vi "EnFlo_TubingCorrection.vi"() -> ()   [LabVIEW 2022 SP3]
uses:
  Globals/Meas_global.vi
  <vilib>/Analysis/NI_AALBase.lvlib
  <vilib>/Analysis/baseanly.llb/Mean (DBL).vi
  <vilib>/gmath/NI_Gmath.lvlib
  Controls/Setup.ctl
panel:
  in  "Correlation Mode":T1(ring)
  in  "Desired Freq Hz":sgl=80.0
  out "Averaging samples":i32=5
  in  "Switch off Tubing Correction?":bool
  out "Correlation Coefficients":string[][](table)
  out "?":dbl[](graph)
  in  "Subtract Mode":T2(ring)
  in  "Reference Instrument":i32(ring) items=["None", "RZ (C0_P00):COM30_Ch 0", "RZ (C0_P01):COM30_Ch 1", "RZ (C0_P02):COM30_Ch 2", "RZ (C0_P03):COM30_Ch 3", "RZ (C0_P04):COM30_Ch 4", "RZ (C0_P05):COM30_Ch 5", "RZ (C0_P06):COM30_Ch 6", "RZ (C0_P07):COM30_Ch 7", "RZ (C0_P10):COM30_Ch 8", "RZ (C0_P11):COM30_Ch 9", "RZ (C0_P12):COM30_Ch 10", "RZ (C0_P13):COM30_Ch 11", "RZ (C0_P14):COM30_Ch 12", "RZ (C0_P15):COM30_Ch 13", "RZ (C0_P16):COM30_Ch 14", "RZ (C0_P17):COM30_Ch 15", "RZ (C0_P20):COM30_Ch 16", "RZ (C0_P21):COM30_Ch 17", "RZ (C0_P22):COM30_Ch 18", "RZ (C0_P23):COM30_Ch 19", "RZ (C0_P24):COM30_Ch 20", "RZ (C0_P25):COM30_Ch 21", "RZ (C0_P26):COM30_Ch 22", "RZ (C0_P27):COM30_Ch 23", "RZ (C0_P30):COM30_Ch 24", "RZ (C0_P31):COM30_Ch 25", "RZ (C0_P32):COM30_Ch 26", "RZ (C0_P33):COM30_Ch 27", "RZ (C0_P34):COM30_Ch 28", "RZ (C0_P35):COM30_Ch 29", "RZ (C0_P36):COM30_Ch 30", "RZ (C0_P37):COM30_Ch 31", "RZ (C0_P40):COM30_Ch 32", "RZ (C0_P41):COM30_Ch 33", "RZ (C0_P42):COM30_Ch 34", "RZ (C0_P43):COM30_Ch 35", "RZ (C0_P44):COM30_Ch 36", "RZ (C0_P45):COM30_Ch 37", "RZ (C0_P46):COM30_Ch 38", "RZ (C0_P47):COM30_Ch 39", "RZ (C0_P50):COM30_Ch 40", "RZ (C0_P51):COM30_Ch 41", "RZ (C1_P73):COM31_Ch 59", "RZ (C0_P53):COM30_Ch 43", "RZ (C0_P54):COM30_Ch 44", "RZ (C0_P55):COM30_Ch 45", "RZ (C0_P56):COM30_Ch 46", "RZ (C0_P57):COM30_Ch 47", "RZ (C0_P60):COM30_Ch 48", "RZ (C0_P62):COM30_Ch 50", "RZ (C0_P63):COM30_Ch 51", "RZ (C0_P64):COM30_Ch 52", "RZ (C0_P65):COM30_Ch 53", "RZ (C0_P66):COM30_Ch 54", "RZ (C0_P67):COM30_Ch 55", "RZ (C0_P70):COM30_Ch 56", "RZ (C0_P71):COM30_Ch 57", "RZ (C0_P72):COM30_Ch 58", "RZ (C0_P73):COM30_Ch 59", "RZ (C0_P74):COM30_Ch 60", "RZ (C0_P75):COM30_Ch 61", "RZ (C0_P76):COM30_Ch 62", "RZ (C0_P77):COM30_Ch 63", "RZ (C1_P00):COM31_Ch 0", "RZ (C1_P01):COM31_Ch 1", "RZ (C1_P02):COM31_Ch 2", "RZ (C1_P03):COM31_Ch 3", "RZ (C1_P04):COM31_Ch 4", "RZ (C1_P05):COM31_Ch 5", "RZ (C1_P06):COM31_Ch 6", "RZ (C1_P07):COM31_Ch 7", "RZ (C1_P10):COM31_Ch 8", "RZ (C1_P11):COM31_Ch 9", "RZ (C1_P12):COM31_Ch 10", "RZ (C1_P13):COM31_Ch 11", "RZ (C1_P14):COM31_Ch 12", "RZ (C1_P15):COM31_Ch 13", "RZ (C1_P16):COM31_Ch 14", "RZ (C1_P17):COM31_Ch 15", "RZ (C1_P20):COM31_Ch 16", "RZ (C1_P21):COM31_Ch 17", "RZ (C1_P22):COM31_Ch 18", "RZ (C1_P23):COM31_Ch 19", "RZ (C1_P24):COM31_Ch 20", "RZ (C1_P25):COM31_Ch 21", "RZ (C1_P26):COM31_Ch 22", "RZ (C1_P27):COM31_Ch 23", "RZ (C1_P30):COM31_Ch 24", "RZ (C1_P31):COM31_Ch 25", "RZ (C1_P32):COM31_Ch 26", "RZ (C1_P33):COM31_Ch 27", "RZ (C1_P34):COM31_Ch 28", "RZ (C1_P35):COM31_Ch 29", "RZ (C1_P36):COM31_Ch 30", "RZ (C1_P37):COM31_Ch 31", "RZ (C1_P40):COM31_Ch 32", "RZ (C1_P41):COM31_Ch 33", "RZ (C1_P42):COM31_Ch 34", "RZ (C1_P43):COM31_Ch 35", "RZ (C1_P44):COM31_Ch 36", "RZ (C1_P45):COM31_Ch 37", "RZ (C1_P46):COM31_Ch 38", "RZ (C1_P47):COM31_Ch 39", "RZ (C1_P50):COM31_Ch 40", "RZ (C1_P51):COM31_Ch 41", "RZ (C1_P52):COM31_Ch 42", "RZ (C1_P53):COM31_Ch 43", "RZ (C1_P54):COM31_Ch 44", "RZ (C1_P55):COM31_Ch 45", "RZ (C1_P56):COM31_Ch 46", "RZ (C1_P57):COM31_Ch 47", "RZ (C1_P60):COM31_Ch 48", "RZ (C1_P61):COM31_Ch 49", "RZ (C1_P62):COM31_Ch 50", "RZ (C1_P63):COM31_Ch 51", "RZ (C2_P00):COM33_Ch 0", "RZ (C2_P01):COM33_Ch 1", "RZ (C2_P02):COM33_Ch 2", "RZ (C2_P03):COM33_Ch 3", "RZ (C2_P04):COM33_Ch 4", "RZ (C2_P05):COM33_Ch 5", "RZ (C2_P06):COM33_Ch 6", "RZ (C2_P07):COM33_Ch 7", "RZ (C2_P10):COM33_Ch 8", "RZ (C2_P11):COM33_Ch 9", "RZ (C2_P12):COM33_Ch 10", "RZ (C2_P13):COM33_Ch 11", "RZ (C2_P14):COM33_Ch 12", "RZ (C2_P15):COM33_Ch 13", "RZ (C2_P16):COM33_Ch 14", "RZ (C2_P17):COM33_Ch 15", "RZ (C2_P20):COM33_Ch 16", "RZ (C2_P21):COM33_Ch 17", "RZ (C2_P22):COM33_Ch 18", "RZ (C2_P23):COM33_Ch 19", "RZ (C2_P24):COM33_Ch 20", "RZ (C2_P25):COM33_Ch 21", "RZ (C2_P26):COM33_Ch 22", "RZ (C2_P27):COM33_Ch 23", "RZ (C2_P31):COM33_Ch 25", "RZ (C2_P32):COM33_Ch 26", "RZ (C2_P33):COM33_Ch 27", "RZ (C2_P34):COM33_Ch 28", "RZ (C2_P35):COM33_Ch 29", "RZ (C2_P36):COM33_Ch 30", "RZ (C2_P37):COM33_Ch 31", "RZ (C2_P40):COM33_Ch 32", "RZ (C2_P41):COM33_Ch 33", "RZ (C2_P42):COM33_Ch 34", "RZ (C2_P43):COM33_Ch 35", "RZ (C2_P44):COM33_Ch 36", "RZ (C2_P45):COM33_Ch 37", "RZ (C2_P46):COM33_Ch 38", "RZ (C2_P47):COM33_Ch 39", "RZ (C2_P50):COM33_Ch 40", "RZ (C2_P51):COM33_Ch 41", "RZ (C2_P52):COM33_Ch 42", "RZ (C2_P53):COM33_Ch 43", "RZ (C2_P54):COM33_Ch 44", "RZ (C2_P55):COM33_Ch 45", "RZ (C2_P56):COM33_Ch 46", "RZ (C2_P57):COM33_Ch 47", "RZ (C2_P60):COM33_Ch 48", "RZ (C2_P61):COM33_Ch 49", "RZ (C2_P62):COM33_Ch 50", "RZ (C2_P63):COM33_Ch 51", "RZ (C2_P64):COM33_Ch 52", "RZ (C2_P65):COM33_Ch 53", "RZ (C2_P66):COM33_Ch 54", "RZ (C2_P67):COM33_Ch 55", "RZ (C2_P70):COM33_Ch 56", "RZ (C2_P71):COM33_Ch 57", "RZ (C2_P72):COM33_Ch 58", "RZ (C2_P73):COM33_Ch 59", "RZ (C2_P74):COM33_Ch 60", "RZ (C2_P75):COM33_Ch 61", "RZ (C2_P76):COM33_Ch 62", "RZ (C2_P77):COM33_Ch 63", "RZ (C3_P00):COM32_Ch 0", "RZ (C3_P01):COM32_Ch 1", "RZ (C3_P02):COM32_Ch 2", "RZ (C3_P03):COM32_Ch 3", "RZ (C3_P04):COM32_Ch 4", "RZ (C3_P05):COM32_Ch 5", "RZ (C3_P06):COM32_Ch 6", "RZ (C3_P07):COM32_Ch 7", "RZ (C3_P10):COM32_Ch 8", "RZ (C3_P11):COM32_Ch 9", "RZ (C3_P12):COM32_Ch 10", "RZ (C3_P13):COM32_Ch 11", "RZ (C3_P14):COM32_Ch 12", "RZ (C3_P15):COM32_Ch 13", "RZ (C3_P16):COM32_Ch 14", "RZ (C3_P17):COM32_Ch 15", "RZ (C3_P20):COM32_Ch 16", "RZ (C3_P21):COM32_Ch 17", "RZ (C3_P22):COM32_Ch 18", "RZ (C3_P23):COM32_Ch 19", "RZ (C3_P24):COM32_Ch 20", "RZ (C3_P25):COM32_Ch 21", "RZ (C3_P26):COM32_Ch 22", "RZ (C3_P27):COM32_Ch 23", "RZ (C3_P30):COM32_Ch 24", "RZ (C3_P31):COM32_Ch 25", "RZ (C3_P33):COM32_Ch 27", "RZ (C3_P34):COM32_Ch 28", "RZ (C3_P35):COM32_Ch 29", "RZ (C3_P36):COM32_Ch 30", "RZ (C3_P37):COM32_Ch 31", "RZ (C3_P40):COM32_Ch 32", "RZ (C3_P41):COM32_Ch 33", "RZ (C3_P42):COM32_Ch 34", "RZ (C3_P43):COM32_Ch 35", "RZ (C3_P44):COM32_Ch 36", "RZ (C3_P45):COM32_Ch 37", "RZ (C3_P46):COM32_Ch 38", "RZ (C3_P47):COM32_Ch 39", "RZ (C3_P50):COM32_Ch 40", "RZ (C3_P51):COM32_Ch 41", "RZ (C3_P52):COM32_Ch 42", "RZ (C3_P53):COM32_Ch 43", "RZ (C3_P54):COM32_Ch 44", "RZ (C3_P55):COM32_Ch 45", "RZ (C3_P56):COM32_Ch 46", "RZ (C3_P60):COM32_Ch 48", "RZ (C3_P61):COM32_Ch 49", "RZ (C3_P62):COM32_Ch 50", "RZ (C3_P63):COM32_Ch 51", "RZ (C3_P64):COM32_Ch 52", "RZ (C3_P65):COM32_Ch 53", "RZ (C3_P66):COM32_Ch 54", "RZ (C3_P70):COM32_Ch 56", "RZ (C3_P71):COM32_Ch 57", "RZ (C3_P72):COM32_Ch 58", "RZ (C3_P73):COM32_Ch 59", "RZ (C3_P74):COM32_Ch 60", "RZ (C3_P75):COM32_Ch 61", "RZ (C3_P77):COM32_Ch 63", "RZ (C4_P00):COM25_Ch 0", "RZ (C4_P01):COM25_Ch 1", "RZ (C4_P02):COM25_Ch 2", "RZ (C4_P03):COM25_Ch 3", "RZ (C4_P04):COM25_Ch 4", "RZ (C4_P05):COM25_Ch 5", "RZ (C4_P06):COM25_Ch 6", "RZ (C4_P07):COM25_Ch 7", "RZ (C4_P10):COM25_Ch 8", "RZ (C4_P11):COM25_Ch 9", "RZ (C4_P12):COM25_Ch 10", "RZ (C4_P13):COM25_Ch 11", "RZ (C4_P15):COM25_Ch 13", "RZ (C4_P16):COM25_Ch 14", "RZ (C4_P17):COM25_Ch 15", "RZ (C4_P20):COM25_Ch 16", "RZ (C4_P21):COM25_Ch 17", "RZ (C4_P22):COM25_Ch 18", "RZ (C4_P23):COM25_Ch 19", "RZ (C4_P24):COM25_Ch 20", "RZ (C4_P26):COM25_Ch 22", "RZ (C4_P27):COM25_Ch 23", "RZ (C4_P30):COM25_Ch 24", "RZ (C4_P32):COM25_Ch 26", "RZ (C4_P33):COM25_Ch 27", "RZ (C4_P34):COM25_Ch 28", "RZ (C4_P35):COM25_Ch 29", "RZ (C4_P36):COM25_Ch 30", "RZ (C4_P37):COM25_Ch 31", "RZ (C4_P40):COM25_Ch 32", "RZ (C4_P41):COM25_Ch 33", "RZ (C4_P42):COM25_Ch 34", "RZ (C4_P43):COM25_Ch 35", "RZ (C4_P44):COM25_Ch 36", "RZ (C4_P45):COM25_Ch 37", "RZ (C4_P46):COM25_Ch 38", "RZ (C4_P47):COM25_Ch 39", "RZ (C4_P50):COM25_Ch 40", "RZ (C4_P51):COM25_Ch 41", "RZ (C4_P52):COM25_Ch 42", "RZ (C4_P53):COM25_Ch 43", "RZ (C4_P54):COM25_Ch 44", "RZ (C4_P55):COM25_Ch 45", "RZ (C4_P56):COM25_Ch 46", "RZ (C4_P57):COM25_Ch 47", "RZ (C4_P60):COM25_Ch 48", "RZ (C4_P61):COM25_Ch 49", "RZ (C4_P62):COM25_Ch 50", "RZ (C4_P63):COM25_Ch 51", "RZ (C4_P64):COM25_Ch 52", "RZ (C4_P65):COM25_Ch 53", "RZ (C4_P66):COM25_Ch 54", "RZ (C4_P67):COM25_Ch 55", "RZ (C4_P70):COM25_Ch 56", "RZ (C4_P71):COM25_Ch 57", "RZ (C4_P72):COM25_Ch 58", "RZ (C4_P73):COM25_Ch 59", "RZ (C4_P74):COM25_Ch 60", "RZ (C4_P75):COM25_Ch 61", "RZ (C4_P76):COM25_Ch 62", "RZ (C4_P77):COM25_Ch 63", "RZ (C5_P00):COM26_Ch 0", "RZ (C5_P01):COM26_Ch 1", "RZ (C5_P02):COM26_Ch 2", "RZ (C5_P03):COM26_Ch 3", "RZ (C5_P04):COM26_Ch 4", "RZ (C5_P05):COM26_Ch 5", "RZ (C5_P06):COM26_Ch 6", "RZ (C5_P07):COM26_Ch 7", "RZ (C5_P10):COM26_Ch 8", "RZ (C5_P11):COM26_Ch 9", "RZ (C5_P12):COM26_Ch 10", "RZ (C5_P13):COM26_Ch 11", "RZ (C5_P14):COM26_Ch 12", "RZ (C5_P15):COM26_Ch 13", "RZ (C5_P16):COM26_Ch 14", "RZ (C5_P17):COM26_Ch 15", "RZ (C5_P20):COM26_Ch 16", "RZ (C5_P21):COM26_Ch 17", "RZ (C5_P22):COM26_Ch 18", "RZ (C5_P23):COM26_Ch 19", "RZ (C5_P24):COM26_Ch 20", "RZ (C5_P25):COM26_Ch 21", "RZ (C5_P26):COM26_Ch 22", "RZ (C5_P27):COM26_Ch 23", "RZ (C5_P30):COM26_Ch 24", "RZ (C5_P31):COM26_Ch 25", "RZ (C5_P32):COM26_Ch 26", "RZ (C5_P33):COM26_Ch 27", "RZ (C5_P34):COM26_Ch 28", "RZ (C5_P35):COM26_Ch 29", "RZ (C5_P36):COM26_Ch 30", "RZ (C5_P37):COM26_Ch 31", "RZ (C5_P40):COM26_Ch 32", "RZ (C5_P41):COM26_Ch 33", "RZ (C5_P42):COM26_Ch 34", "RZ (C5_P43):COM26_Ch 35", "RZ (C5_P44):COM26_Ch 36", "RZ (C5_P45):COM26_Ch 37", "RZ (C5_P46):COM26_Ch 38", "RZ (C5_P47):COM26_Ch 39", "RZ (C5_P50):COM26_Ch 40", "RZ (C5_P51):COM26_Ch 41", "RZ (C5_P52):COM26_Ch 42", "RZ (C5_P53):COM26_Ch 43", "RZ (C5_P54):COM26_Ch 44", "RZ (C5_P55):COM26_Ch 45", "RZ (C5_P56):COM26_Ch 46", "RZ (C5_P60):COM26_Ch 48", "RZ (C5_P61):COM26_Ch 49", "RZ (C5_P62):COM26_Ch 50", "RZ (C5_P63):COM26_Ch 51", "RZ (C5_P64):COM26_Ch 52", "RZ (C5_P65):COM26_Ch 53", "RZ (C5_P66):COM26_Ch 54", "RZ (C5_P67):COM26_Ch 55", "RZ (C5_P71):COM26_Ch 57", "RZ (C5_P72):COM26_Ch 58", "RZ (C5_P73):COM26_Ch 59", "RZ (C5_P74):COM26_Ch 60", "RZ (C5_P75):COM26_Ch 61", "RZ (C5_P76):COM26_Ch 62", "RZ (C5_P77):COM26_Ch 63", "RZ (C6_P02):COM28_Ch 2", "RZ (C6_P03):COM28_Ch 3", "RZ (C6_P04):COM28_Ch 4", "RZ (C6_P05):COM28_Ch 5", "RZ (C6_P06):COM28_Ch 6", "RZ (C6_P07):COM28_Ch 7", "RZ (C6_P12):COM28_Ch 10", "RZ (C6_P13):COM28_Ch 11", "RZ (C6_P14):COM28_Ch 12", "RZ (C6_P15):COM28_Ch 13", "RZ (C6_P16):COM28_Ch 14", "RZ (C6_P17):COM28_Ch 15", "RZ (C6_P20):COM28_Ch 16", "RZ (C6_P21):COM28_Ch 17", "RZ (C6_P22):COM28_Ch 18", "RZ (C6_P23):COM28_Ch 19", "RZ (C6_P24):COM28_Ch 20", "RZ (C6_P25):COM28_Ch 21", "RZ (C6_P26):COM28_Ch 22", "RZ (C6_P27):COM28_Ch 23", "RZ (C6_P30):COM28_Ch 24", "RZ (C6_P31):COM28_Ch 25", "RZ (C6_P32):COM28_Ch 26", "RZ (C6_P33):COM28_Ch 27", "RZ (C6_P34):COM28_Ch 28", "RZ (C6_P35):COM28_Ch 29", "RZ (C6_P36):COM28_Ch 30", "RZ (C6_P37):COM28_Ch 31", "RZ (C6_P40):COM28_Ch 32", "RZ (C6_P41):COM28_Ch 33", "RZ (C6_P42):COM28_Ch 34", "RZ (C6_P43):COM28_Ch 35", "RZ (C6_P44):COM28_Ch 36", "RZ (C6_P45):COM28_Ch 37", "RZ (C6_P46):COM28_Ch 38", "RZ (C6_P47):COM28_Ch 39", "RZ (C6_P50):COM28_Ch 40", "RZ (C6_P51):COM28_Ch 41", "RZ (C6_P52):COM28_Ch 42", "RZ (C6_P53):COM28_Ch 43", "RZ (C6_P54):COM28_Ch 44", "RZ (C6_P55):COM28_Ch 45", "RZ (C6_P56):COM28_Ch 46", "RZ (C6_P60):COM28_Ch 48", "RZ (C6_P61):COM28_Ch 49", "RZ (C6_P62):COM28_Ch 50", "RZ (C6_P63):COM28_Ch 51", "RZ (C6_P64):COM28_Ch 52", "RZ (C6_P65):COM28_Ch 53", "RZ (C6_P66):COM28_Ch 54", "RZ (C6_P67):COM28_Ch 55", "RZ (C6_P70):COM28_Ch 56", "RZ (C6_P71):COM28_Ch 57", "RZ (C6_P72):COM28_Ch 58", "RZ (C6_P73):COM28_Ch 59", "RZ (C6_P74):COM28_Ch 60", "RZ (C6_P75):COM28_Ch 61", "RZ (C6_P76):COM28_Ch 62", "RZ (C6_P77):COM28_Ch 63", "RZ (C7_P00):COM27_Ch 0", "RZ (C7_P01):COM27_Ch 1", "RZ (C7_P02):COM27_Ch 2", "RZ (C7_P03):COM27_Ch 3", "RZ (C7_P04):COM27_Ch 4", "RZ (C7_P05):COM27_Ch 5", "RZ (C7_P06):COM27_Ch 6", "RZ (C7_P07):COM27_Ch 7", "RZ (C7_P10):COM27_Ch 8", "RZ (C7_P11):COM27_Ch 9", "RZ (C7_P12):COM27_Ch 10", "RZ (C7_P13):COM27_Ch 11", "RZ (C7_P14):COM27_Ch 12", "RZ (C7_P15):COM27_Ch 13", "RZ (C7_P16):COM27_Ch 14", "RZ (C7_P17):COM27_Ch 15", "RZ (C7_P20):COM27_Ch 16", "RZ (C7_P21):COM27_Ch 17", "RZ (C7_P22):COM27_Ch 18", "RZ (C7_P23):COM27_Ch 19", "RZ (C7_P24):COM27_Ch 20", "RZ (C7_P25):COM27_Ch 21", "RZ (C7_P26):COM27_Ch 22", "RZ (C7_P27):COM27_Ch 23", "RZ (C7_P30):COM27_Ch 24", "RZ (C7_P31):COM27_Ch 25", "RZ (C7_P32):COM27_Ch 26", "RZ (C7_P33):COM27_Ch 27", "RZ (C7_P34):COM27_Ch 28", "RZ (C7_P35):COM27_Ch 29", "RZ (C7_P36):COM27_Ch 30", "RZ (C7_P37):COM27_Ch 31", "RZ (C7_P40):COM27_Ch 32", "RZ (C7_P41):COM27_Ch 33", "RZ (C7_P42):COM27_Ch 34", "RZ (C7_P43):COM27_Ch 35", "RZ (C7_P44):COM27_Ch 36", "RZ (C7_P45):COM27_Ch 37", "RZ (C7_P46):COM27_Ch 38", "RZ (C7_P47):COM27_Ch 39", "RZ (C7_P50):COM27_Ch 40", "RZ (C7_P51):COM27_Ch 41", "RZ (C7_P52):COM27_Ch 42", "RZ (C7_P53):COM27_Ch 43", "RZ (C7_P54):COM27_Ch 44", "RZ (C7_P55):COM27_Ch 45", "RZ (C7_P56):COM27_Ch 46", "RZ (C7_P57):COM27_Ch 47", "RZ (C7_P60):COM27_Ch 48", "RZ (C7_P61):COM27_Ch 49", "RZ (C7_P62):COM27_Ch 50", "RZ (C7_P63):COM27_Ch 51", "RZ (C7_P64):COM27_Ch 52", "RZ (C7_P65):COM27_Ch 53", "RZ (C7_P66):COM27_Ch 54", "RZ (C7_P67):COM27_Ch 55", "RZ (C7_P70):COM27_Ch 56", "RZ (C7_P71):COM27_Ch 57", "RZ (C7_P72):COM27_Ch 58", "RZ (C7_P73):COM27_Ch 59", "RZ (C7_P74):COM27_Ch 60", "RZ (C7_P75):COM27_Ch 61", "RZ (C7_P76):COM27_Ch 62", "RZ (C7_P77):COM27_Ch 63", "FF (C):COM13_Ch 1", "FF (Cref):COM13_Ch 2"]
  in  "Select Freq Calib file":path
  in  "Calibration File String":string="Joy_13thMay_xls"
  # "Run this vi as a top level to inject setup information into either a Measurement Setup File or Raw Data files."
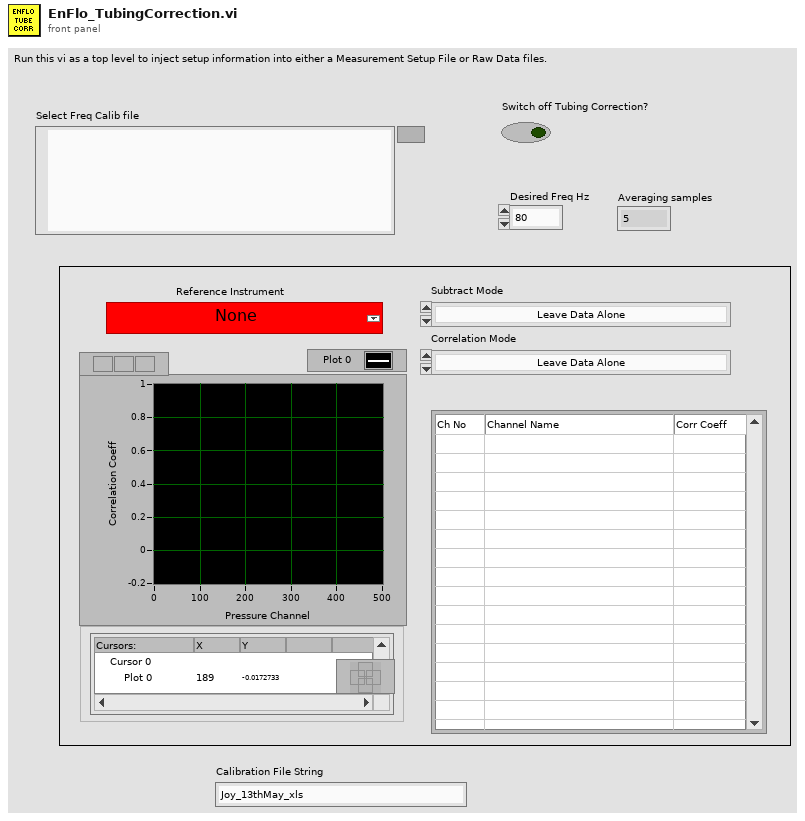
[diagram p1: front panel]
types:
  T1 = enum16{"Leave Data Alone", "Correlate with Ref Channel"}
  T2 = enum16{"Leave Data Alone", "Subtract Ref Channel", "Subtract Instantaneous Average of All Chs"}
  T3 = typedef "Setup.ctl" = enum16{"Run Program", "Show Setup", "Save Current Setup", "Setup Front Panel"}
  T4 = typedef "Analysis_info_cluster.ctl" = cluster{"Colour":u32, "Inst type":T5, "Inst name":string, "Symbol":string, "Code name":string, "Extra Info":string, "Inst Array":T6, "U":dbl, "u^2":dbl, "u^3":dbl, "u^4":dbl, "Skew_u":dbl, "Kurt_u":dbl, "Sd Error in Mean":dbl, "% u'/U":dbl, "X":dbl, "Y":dbl, "Z":dbl, "Timescale integral Estimate":dbl, "Sd Error in Variance":dbl, "Calib File":path, "Calib Constants":dbl[], "Output Position":bool, "Stats":enum16{"None", "Basic", "Full"}, "Av Sampling Rate":dbl, "Av No of Samples":dbl, "Total Meas Time (s)":dbl, "OrigChName":string, "Max value":dbl, "Min value":dbl, "Req Sample Rate Hz":dbl, "Sync Delay Time (s)":dbl, "Ch No":i16, "Device":string, "Use Latest Calib":bool, "Port":string, "Metadata Ch Names":string[], "Metadata Ch Values":string[], "Label":string, "chState":T7, "Point Drift":dbl, "inputConfig":string}
  T5 = typedef "Inst_type.ctl" = enum16{"Raw voltage", "Raw with zero offsetting", "Propeller anemometer", "Pressure Transducer", "Pitot-static tube", "Hot wire", "Cross wire 1", "Cross wire 2", "Generic Linear", "Generic Polynomial", "Generic BackPoly", "Fast FID", "Thermocouple", "Cold wire", "Pulsed Wire", "LDA Vel", "LDA Tran time", "LDA Arr time", "Microphone"}
  T6 = typedef "Instrument_Array.ctl" = enum16{"PWA", "LDA", "Analogue"}
  T7 = typedef "channelState.ctl" = enum32{"No Selection", "Solo", "Mute"}
  T8 = typedef "Time_Trace_Cluster.ctl" = cluster{"Weighting":dbl[], "Voltage":dbl[], "Eng Values":dbl[]}
  T9 = typedef "Resample mode.ctl" = cluster{"Mode":enum16{"Index", "Interpolate"}, "Index":dbl[]}
  T10 = typedef "Post_Process.ctl" = enum16{"Take New Data", "Post Process Raw Data File"}
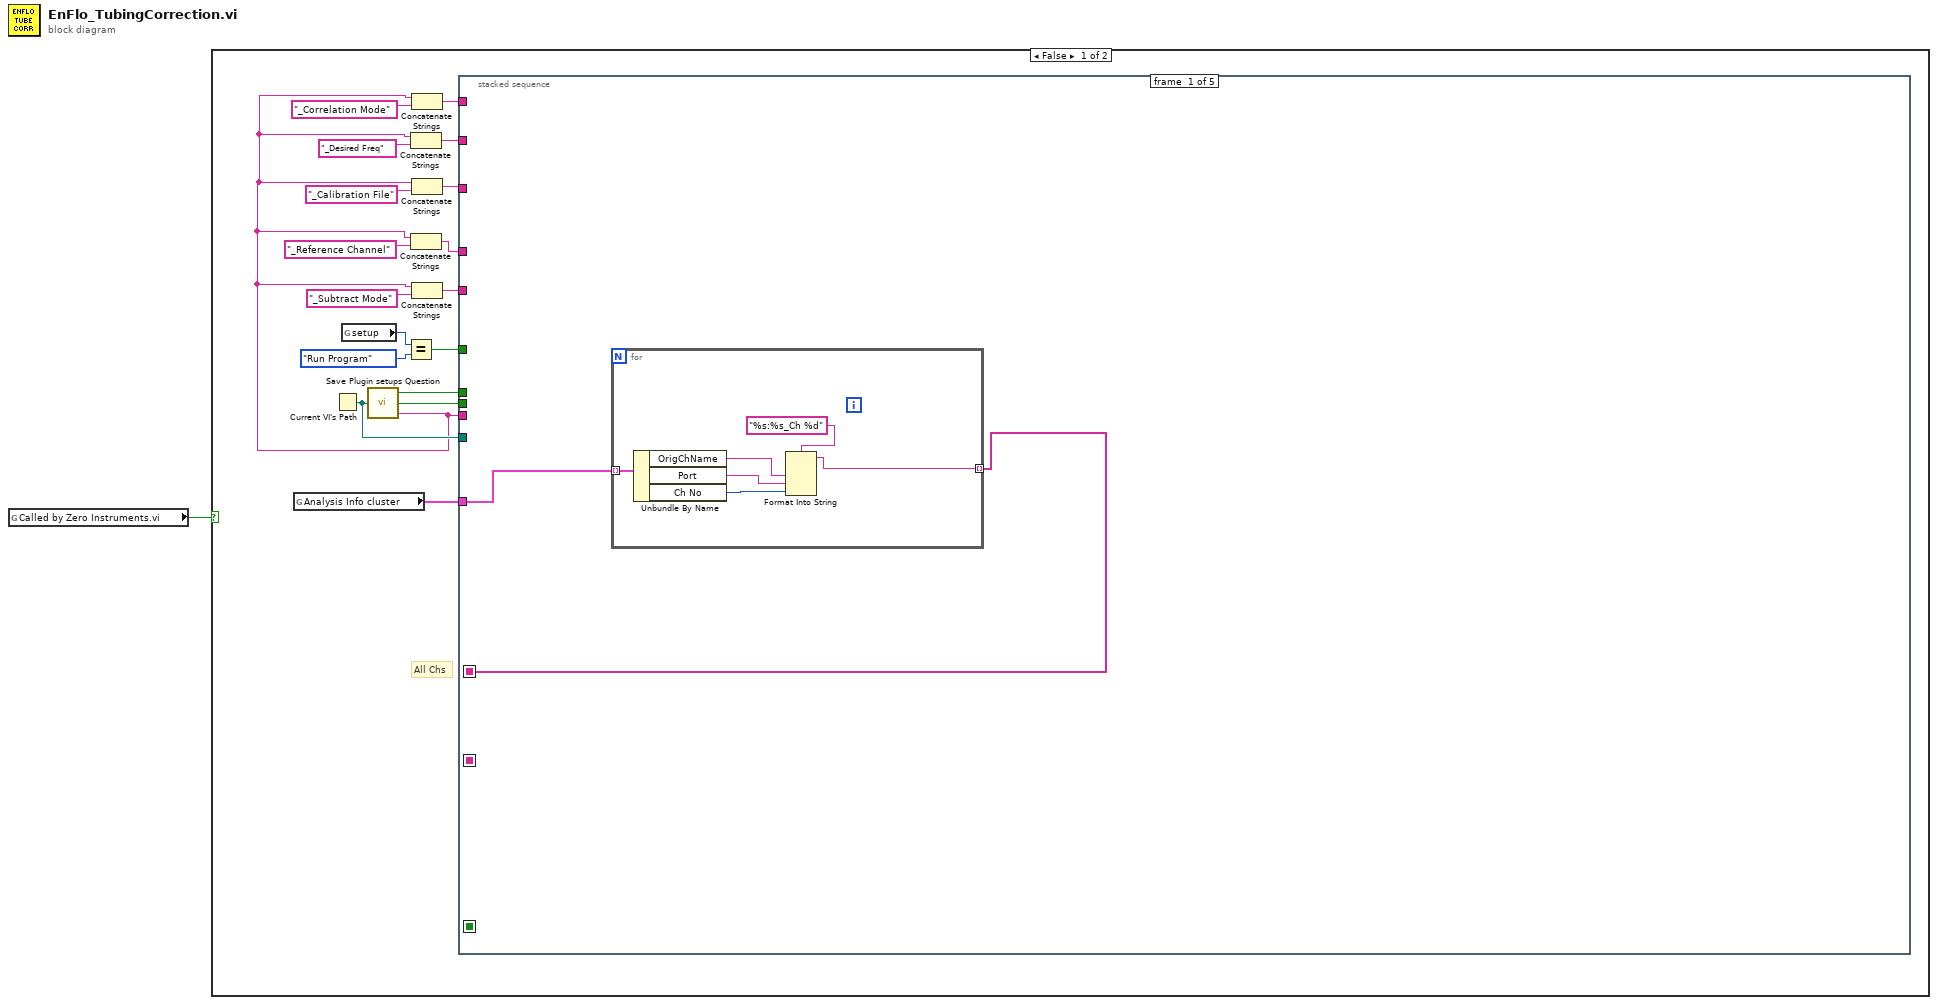
[diagram p0: block diagram]
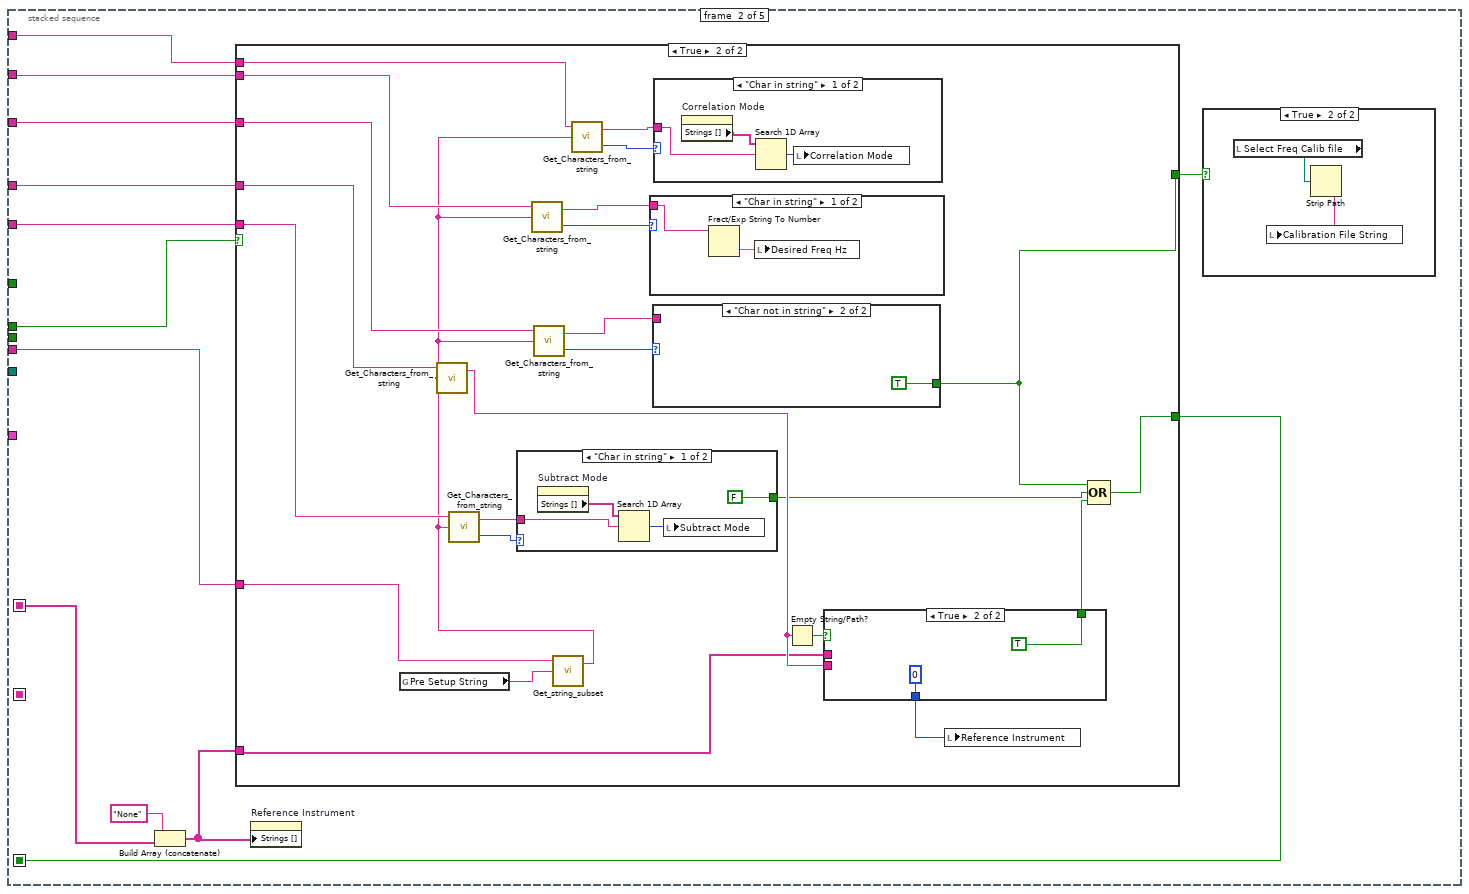
[diagram p2: hidden frame]
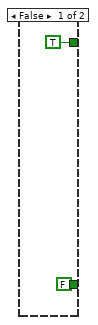
[diagram p4: hidden frame]
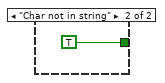
[diagram p7: hidden frame]
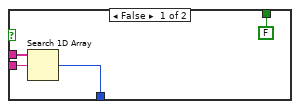
[diagram p8: hidden frame]
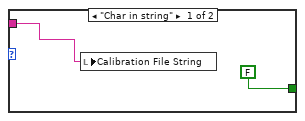
[diagram p9: hidden frame]
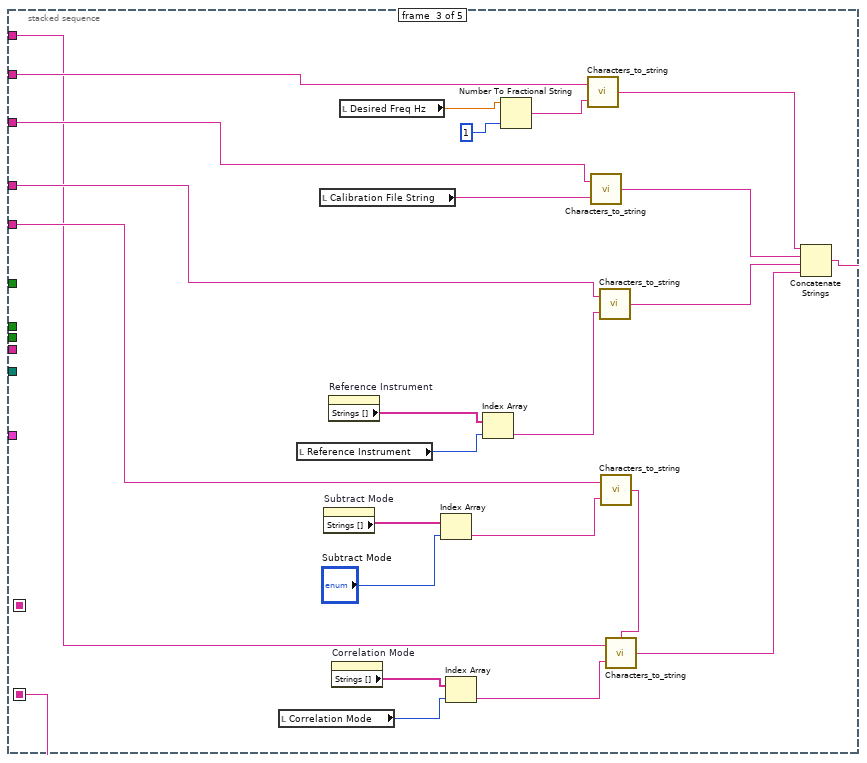
[diagram p10: hidden frame]
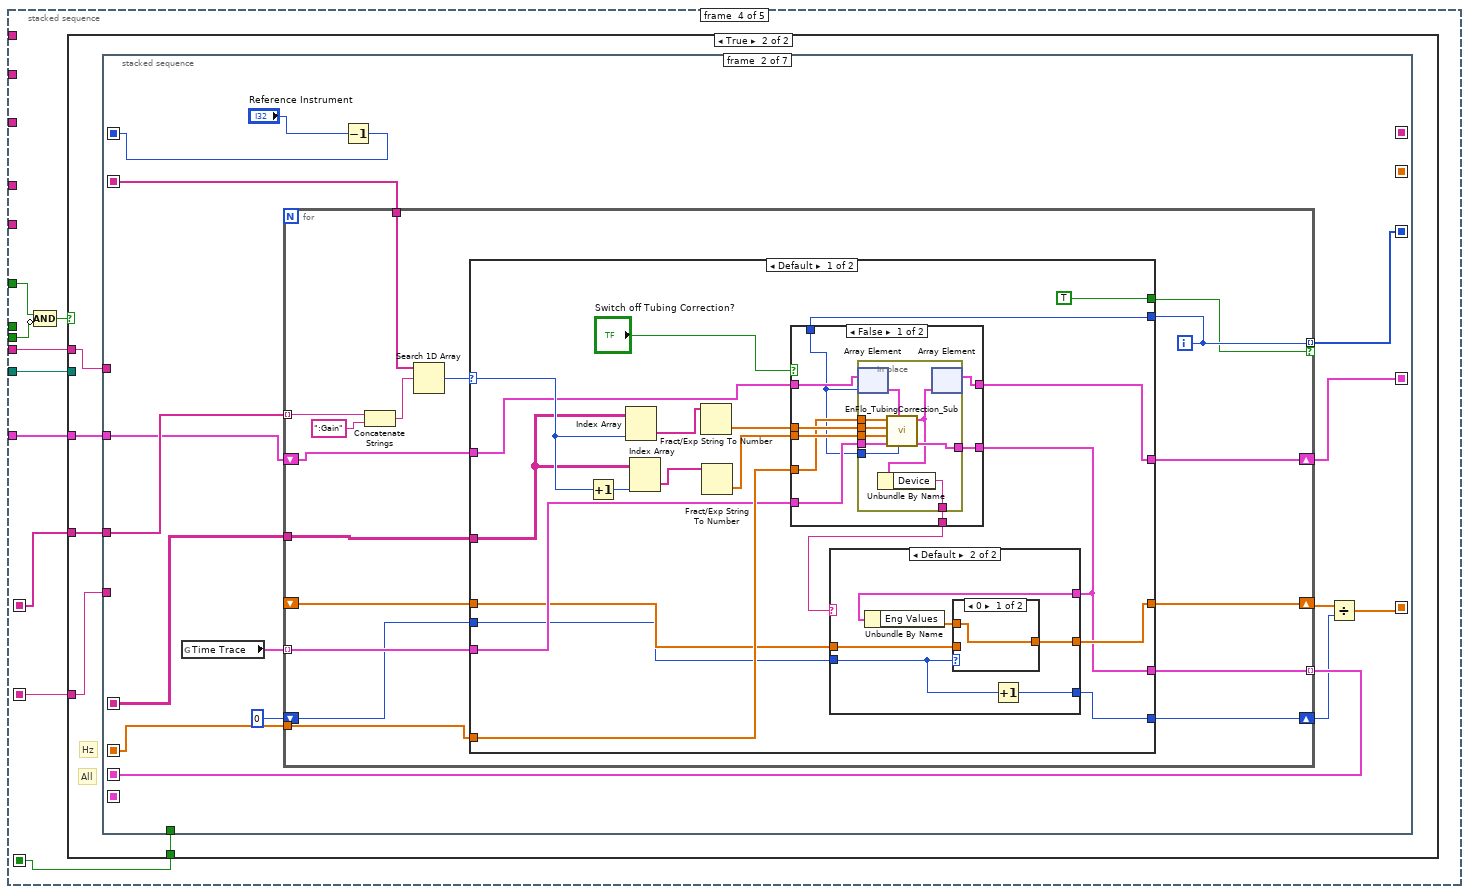
[diagram p11: hidden frame]
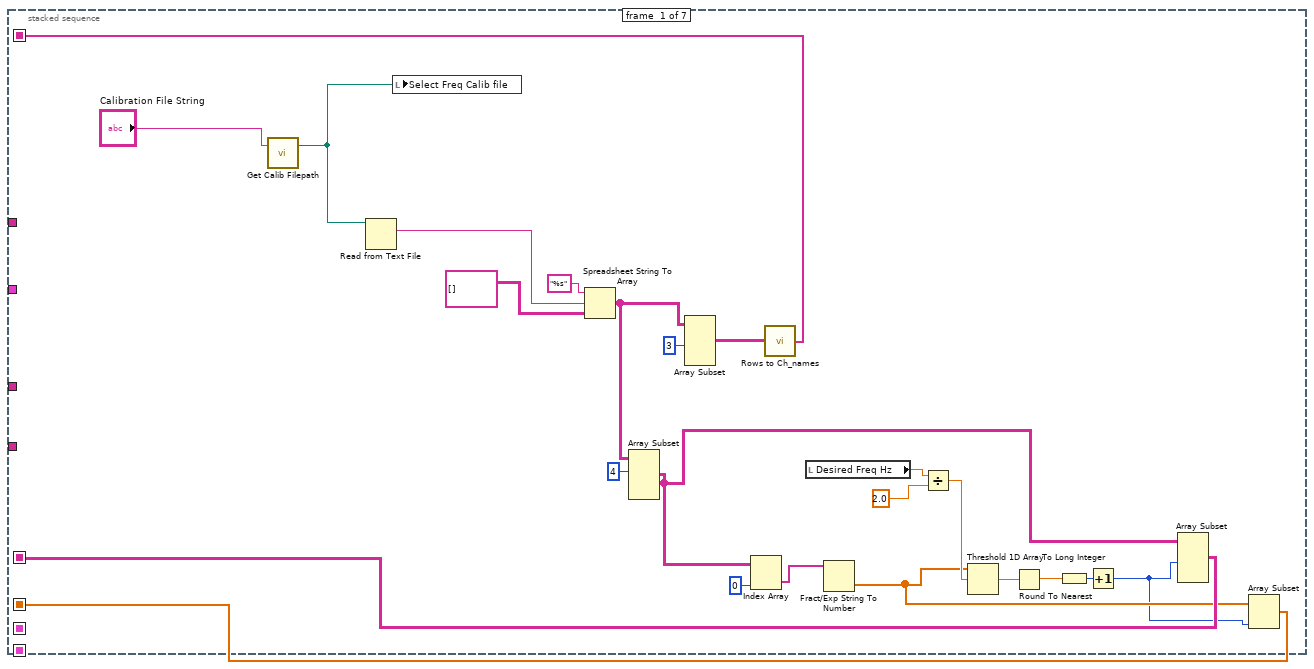
[diagram p13: hidden frame]
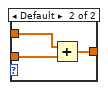
[diagram p15: hidden frame]
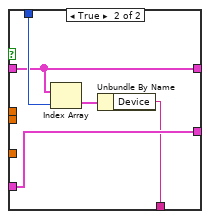
[diagram p16: hidden frame]
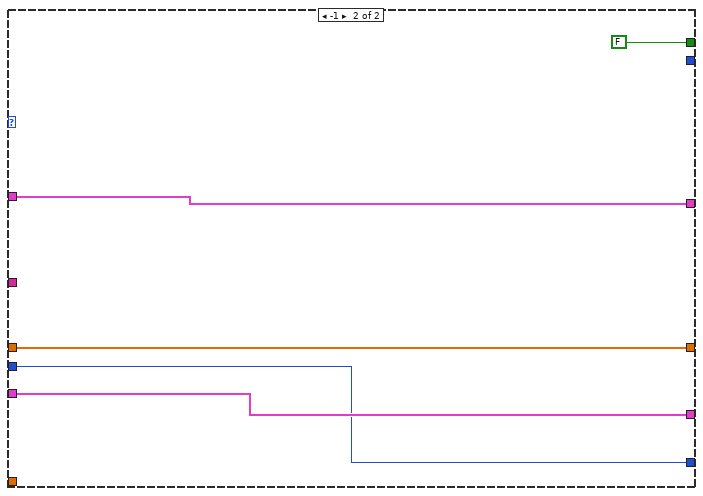
[diagram p17: hidden frame]
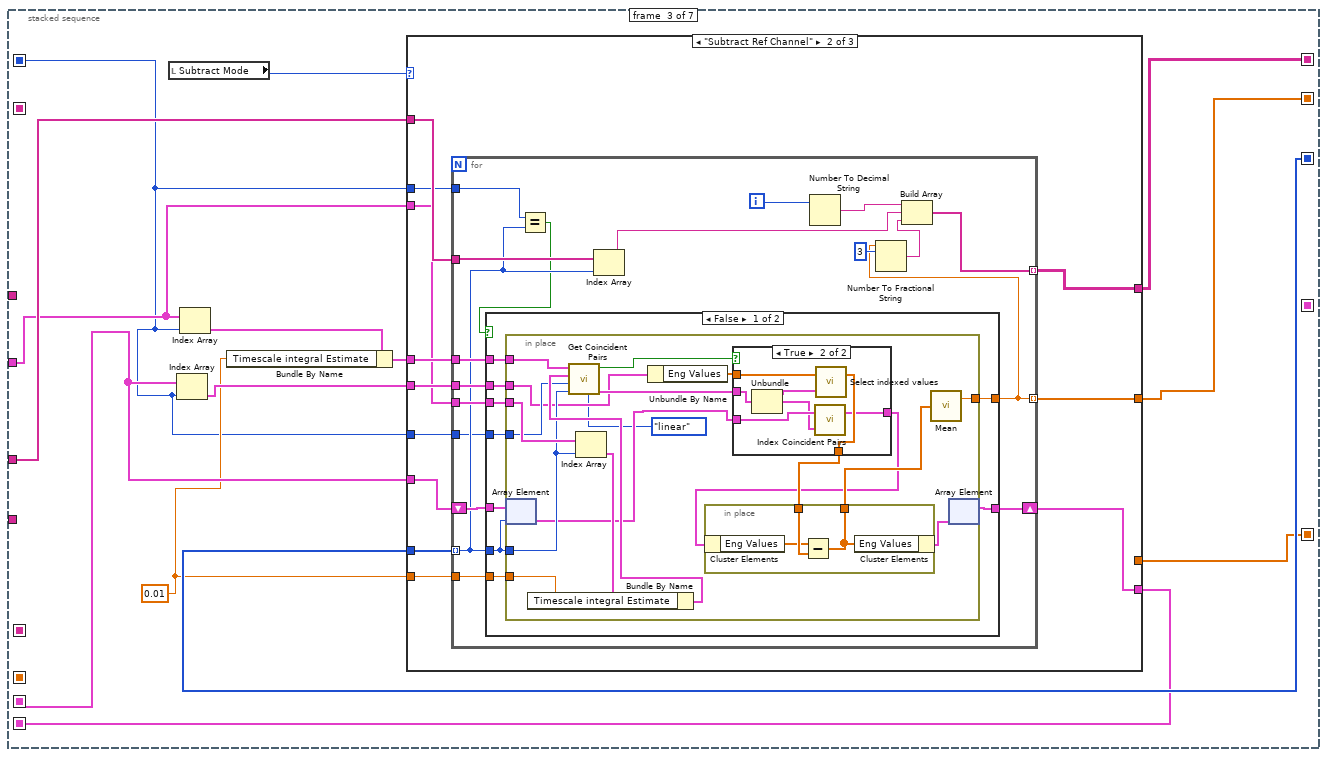
[diagram p18: hidden frame]
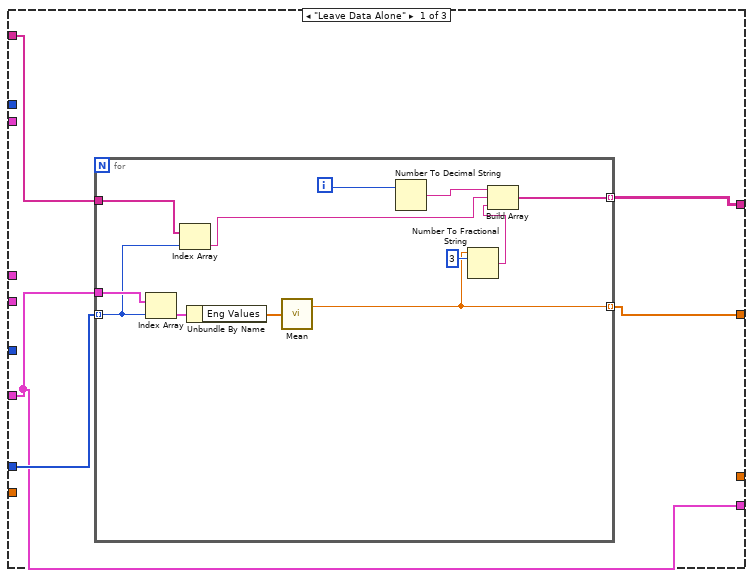
[diagram p19: hidden frame]
diagram:
  n1 = global read "Meas_global.vi" "Called by Zero Instruments.vi"() -> (w1:bool)
  n2 = case shown="False" w1 {
    frame False {
      # "All Chs"
      n3 = global read "Meas_global.vi" "Analysis Info cluster"() -> (w14:T4[])
      n4 = Current VI's Path() -> (path=w15:path)
      n5 = global read "Meas_global.vi" "setup"() -> (w9:T3)
      n6 = call "Save Plugin setups Question.vi"("VI path"=w15) -> ("Load Plugin Setup"=w19:bool, "Save Plugin Setup"=w16:bool, "Plugin_Label"=w3:string)
      n7 = Equal?(x=w9, y=Setup."Run Program" ("setup")) -> (x = y?=w7:bool)
      n8 = Concatenate Strings(w3, "_Desired Freq" ("string")) -> (w5:string)
      n9 = Concatenate Strings(w3, "_Reference Channel" ("string")) -> (w12:string)
      n10 = Concatenate Strings(w3, "_Correlation Mode" ("string")) -> (w2:string)
      n11 = Concatenate Strings(w3, "_Calibration File" ("string")) -> (w17:string)
      n12 = Concatenate Strings(w3, "_Subtract Mode" ("string")) -> (w10:string)
      n13 = stacked-sequence {
        seq-local: [w20 _ _ _ _] -> [_ w33 _ w116 _]
        seq-local: [_ _ w101 _ _] -> [_ _ _ w115 w551]
        seq-local: [_ w31 _ _ _] -> [_ _ _ w114 w550]
        tunnel: w19 -> [_ w39 _ _ _]
        tunnel: w3 -> [_ w38 _ w119 w553]
        tunnel: w17 -> [_ w37 w104 _ _]
        tunnel: w16 -> [_ _ _ w113 w554]
        tunnel: w15 -> [_ _ _ w118 w552]
        tunnel: w14 -> [w21 _ _ w117 _]
        tunnel: w12 -> [_ w36 w103 _ _]
        tunnel: w10 -> [_ w35 w102 _ _]
        tunnel: w7 -> [_ _ _ w112 _]
        tunnel: w5 -> [_ w29 w97 _ _]
        tunnel: w2 -> [_ w28 w89 _ _]
        frame #0 {
          n14 = for {
            tunnel: w21 -> [w25] mode=indexing
            tunnel: [w22] -> w20 mode=indexing
            n15 = Unbundle By Name(w25) -> ("OrigChName"=w24:string, "Port"=w26:string, "Ch No"=w27:i16)
            n16 = Format Into String(format string="%s:%s_Ch %d", w24, w26, w27) -> (resulting string=w22:string)  [unwired: 2 in, 1 out]
          }
        }
        frame #1 {
          n17 = Build Array (concatenate)("None", w33) -> (w32:string[])
          n18 = case shown="True" w39 {
            tunnel: w38 -> [_ w66]
            tunnel: w37 -> [_ w65]
            tunnel: w36 -> [_ w62]
            tunnel: w35 -> [_ w61]
            tunnel: w32 -> [_ w57]
            tunnel: [FALSE w52] -> w31
            tunnel: [TRUE w51] -> w30
            tunnel: w29 -> [_ w48]
            tunnel: w28 -> [_ w45]
            frame False {
            }
            frame True {
              n19 = global read "Meas_global.vi" "Pre Setup String"() -> (w67:string)
              n20 = call "Get_string_subset.vi"("String to split"=w67, "File Label"=w66) -> ("Output string"=w44:string)  [unwired: 2 in, 1 out]
              n21 = call "Get_Characters_from_string.vi"("Input string"=w44, "Variable name"=w62) -> ("Value"=w58:string)  [unwired: 1 in, 1 out]
              n22 = call "Get_Characters_from_string.vi"("Input string"=w44, "Variable name"=w61) -> ("Status"=w55:enum16{"Char in string", "Char not in string"}, "Value"=w60:string)  [unwired: 1 in]
              n23 = case shown="\"Char in string\"" w55 {
                tunnel: w60 -> [w75 _]
                tunnel: [FALSE TRUE] -> w54
                frame "Char in string" {
                  n24 = property on="Subtract Mode" class="Enum (strict)"() -> ("Strings []"=w76:string[])  [unwired: 2 in, 2 out]
                  n25 = Search 1D Array(1D array=w76, element=w75) -> (index of element=w74:i32)  [unwired: 1 out]
                  n26 = local write "Subtract Mode"(w74) -> ()
                }
                frame "Char not in string" {
                }
              }
              n27 = call "Get_Characters_from_string.vi"("Input string"=w44, "Variable name"=w48) -> ("Status"=w49:enum16{"Char in string", "Char not in string"}, "Value"=w50:string)  [unwired: 1 in]
              n28 = call "Get_Characters_from_string.vi"("Input string"=w44, "Variable name"=w65) -> ("Status"=w64:enum16{"Char in string", "Char not in string"}, "Value"=w63:string)  [unwired: 1 in]
              n29 = call "Get_Characters_from_string.vi"("Input string"=w44, "Variable name"=w45) -> ("Status"=w47:enum16{"Char in string", "Char not in string"}, "Value"=w46:string)  [unwired: 1 in]
              n30 = case shown="\"Char in string\"" w49 {
                tunnel: w50 -> [w72 _]
                frame "Char in string" {
                  n31 = Fract/Exp String To Number(string=w72) -> (number=w71:dbl)  [unwired: 3 in, 1 out]
                  n32 = local write "Desired Freq Hz"(w71) -> ()
                }
                frame "Char not in string" {
                }
              }
              n33 = case shown="\"Char not in string\"" w64 {
                tunnel: w63 -> [w85 _]
                tunnel: [FALSE TRUE] -> w51
                frame "Char in string" {
                  n34 = local write "Calibration File String"(w85) -> ()
                }
                frame "Char not in string" {
                }
              }
              n35 = case shown="\"Char in string\"" w47 {
                tunnel: w46 -> [w70 _]
                frame "Char in string" {
                  n36 = property on="Correlation Mode" class="Enum (strict)"() -> ("Strings []"=w68:string[])  [unwired: 2 in, 2 out]
                  n37 = Search 1D Array(1D array=w68, element=w70) -> (index of element=w69:i32)  [unwired: 1 out]
                  n38 = local write "Correlation Mode"(w69) -> ()
                }
                frame "Char not in string" {
                }
              }
              n39 = Empty String/Path?(string/path=w58) -> (empty?=w59:bool)
              n40 = case shown="True" w59 {
                tunnel: w57 -> [w81 _]
                tunnel: w58 -> [w80 _]
                tunnel: [w79 0 ("index of element")] -> w56
                tunnel: [FALSE TRUE] -> w53
                frame False {
                  n41 = Search 1D Array(1D array=w81, element=w80) -> (index of element=w79:i32)  [unwired: 1 out]
                }
                frame True {
                }
              }
              n42 = local write "Reference Instrument"(w56) -> ()
              n43 = Compound Arithmetic op=OR(w51, w54, w53) -> (w52:bool)
            }
          }
          n44 = property on="Reference Instrument" class="Ring (strict)"("Strings []"=w32) -> ()  [unwired: 2 in, 2 out]
          n45 = case shown="True" w30 {
            frame False {
            }
            frame True {
              n46 = local read "Select Freq Calib file"() -> (w41:path)
              n47 = Strip Path(path=w41) -> (name=w40:string)  [unwired: 1 out]
              n48 = local write "Calibration File String"(w40) -> ()
            }
          }
        }
        frame #2 {
          n49 = local read "Correlation Mode"() -> (w90:T1)
          n50 = local read "Reference Instrument"() -> (w107:i32)
          n51 = local read "Calibration File String"() -> (w110:string)
          n52 = property on="Subtract Mode" class="Enum (strict)"() -> ("Strings []"=w99:string[])  [unwired: 2 in, 2 out]
          n53 = property on="Reference Instrument" class="Ring (strict)"() -> ("Strings []"=w106:string[])  [unwired: 2 in, 2 out]
          n54 = property on="Correlation Mode" class="Enum (strict)"() -> ("Strings []"=w91:string[])  [unwired: 2 in, 2 out]
          n55 = local read "Desired Freq Hz"() -> (w96:sgl)
          n56 = Index Array(array=w99, index="Subtract Mode") -> (element=w98:string)
          n57 = Index Array(array=w91, index=w90) -> (element=w92:string)
          n58 = Index Array(array=w106, index=w107) -> (element=w105:string)
          n59 = Number To Fractional String(number=w96, precision (6)=i16 1) -> (F-format string=w95:string)  [unwired: 2 in]
          n60 = call "Characters_to_string.vi"("Characters to write"=w95, "Label for characters"=w97) -> ("Output string"=w93:string)  [unwired: 1 in]
          n61 = call "Characters_to_string.vi"("Characters to write"=w110, "Label for characters"=w104) -> ("Output string"=w108:string)  [unwired: 1 in]
          n62 = call "Characters_to_string.vi"("Characters to write"=w105, "Label for characters"=w103) -> ("Output string"=w109:string)  [unwired: 1 in]
          n63 = call "Characters_to_string.vi"("Characters to write"=w98, "Label for characters"=w102) -> ("Output string"=w88:string)  [unwired: 1 in]
          n64 = call "Characters_to_string.vi"("stringIn"=w88, "Characters to write"=w92, "Label for characters"=w89) -> ("Output string"=w87:string)
          n65 = Concatenate Strings(w93, w108, w109, w87) -> (w101:string)
        }
        frame #3 {
          n66 = Compound Arithmetic op=AND(w112, invert w113) -> (w111:bool)
          n67 = case shown="True" w111 {
            tunnel: w119 -> [_ w122]
            tunnel: w118 -> [_ _]
            tunnel: w117 -> [_ w124]
            tunnel: w116 -> [_ w123]
            tunnel: w115 -> [_ w121]
            tunnel: w114 -> [_ w120]
            frame False {
            }
            frame True {
              # "All"
              # "Hz"
              n68 = stacked-sequence {
                seq-local: [w142 _ _ _ _ _ _] -> [_ w162 _ _ _ _ _]
                seq-local: [w129 _ _ _ _ _ _] -> [_ w161 _ _ _ _ _]
                seq-local: [w126 _ _ _ _ _ _] -> [_ w160 _ _ _ _ _]
                seq-local: [_ w158 _ _ _ _ _] -> [_ _ w253 _ _ _ _]
                seq-local: [_ w157 _ _ _ _ _] -> [_ _ w252 w421 w501 _ _]
                seq-local: [_ w154 _ _ _ _ _] -> [_ _ w240 w419 _ _ _]
                seq-local: [_ w149 _ _ _ _ _] -> [_ _ w249 _ _ _ _]
                seq-local: [_ _ w243 _ _ _ _] -> [_ _ _ w418 w500 _ _]
                seq-local: [_ w148 _ _ _ _ _] -> [_ _ _ w417 _ _ _]
                seq-local: [_ _ w242 _ _ _ _] -> [_ _ _ w413 _ _ _]
                seq-local: [_ _ w241 _ _ _ _] -> [_ _ _ w406 _ _ _]
                tunnel: w124 -> [_ w153 w250 w420 _ _ _]
                tunnel: w123 -> [_ w156 w251 _ _ _ _]
                tunnel: w122 -> [_ _ _ _ _ _ w545]
                tunnel: w121 -> [_ _ _ _ _ _ w544]
                tunnel: w120 -> [_ _ _ _ _ _ w543]
                frame #0 {
                  n69 = call "Get Calib Filepath.vi"("Filename String"="Calibration File String") -> ("Filename Out"=w137:path)  [unwired: 2 in]
                  n70 = Read from Text File(file (use dialog)=w137) -> (text=w145:string)  [unwired: 3 in, 3 out]
                  n71 = local write "Select Freq Calib file"(w137) -> ()
                  n72 = Spreadsheet String To Array(format string="%s", spreadsheet string=w145, array type (2D Dbl)=string[][] []) -> (array=w140:string[][])  [unwired: 1 in]
                  n73 = Array Subset(array=w140, index (row)=4 ("index")) -> (w130:string[][])  [unwired: 3 in]
                  n74 = Array Subset(array=w140, length (row)=3 ("length")) -> (w143:string[][])  [unwired: 3 in]
                  n75 = Index Array(array=w130, index (col)=0 ("disabled index (col)")) -> (element=w138:string[])  [unwired: 1 in]
                  n76 = call "Rows to Ch_names.vi"("array type (2D Dbl)"=w143) -> ("Array"=w142:string[])
                  n77 = local read "Desired Freq Hz"() -> (w135:sgl)
                  n78 = Fract/Exp String To Number(string=w138) -> (number=w128:dbl[])  [unwired: 3 in, 1 out]
                  n79 = Divide(x=w135, y=sgl 2.0) -> (x/y=w133:sgl)
                  n80 = Threshold 1D Array(2:w133, 3:w128) -> (0:w132:dbl)  [unwired: 1 in]
                  n81 = Round To Nearest(number=w132) -> (nearest integer value=w131:dbl)
                  n82 = To Long Integer(number=w131) -> (32bit integer=w127:i32)
                  n83 = Increment(x=w127) -> (x+1=w125:i32)
                  n84 = Array Subset(array=w130, length (row)=w125) -> (w129:string[][])  [unwired: 3 in]
                  n85 = Array Subset(array=w128, length=w125) -> (w126:dbl[])  [unwired: 1 in]
                }
                frame #1 {
                  n86 = global read "Meas_global.vi" "Time Trace"() -> (w159:T8[])
                  n87 = for {
                    tunnel: w162 -> [w171]
                    tunnel: w161 -> [w176]
                    tunnel: w160 -> [w175]
                    tunnel: w159 -> [w174] mode=indexing
                    tunnel: [w173] -> w158 mode=indexing
                    tunnel: [w168] -> w157 mode=indexing if=w163
                    tunnel: w156 -> [w172] mode=indexing
                    shift-right: [w169] -> w148
                    shift-left: w153 -> [w170]
                    shift-right: [w164] -> w150
                    shift-left: 0 -> [w165]
                    shift-right: [w166] -> w151
                    shift-left: _ -> [w167]
                    i -> [w168]
                    n88 = Concatenate Strings(w172, ":Gain" ("string")) -> (w178:string)
                    n89 = Search 1D Array(1D array=w171, element=w178) -> (index of element=w177:i32)  [unwired: 1 out]
                    n90 = case shown="Default" w177 {
                      selector: w177 -> [w198 _]
                      tunnel: w176 -> [w197 _]
                      tunnel: w175 -> [w192 _]
                      tunnel: w174 -> [w190 w239]
                      tunnel: [w183 w239] -> w173
                      tunnel: [TRUE FALSE] -> w163
                      tunnel: w170 -> [w188 w237]
                      tunnel: [w187 w237] -> w169
                      tunnel: w168 -> [w186 _]
                      tunnel: w167 -> [w185 w236]
                      tunnel: [w184 w236] -> w166
                      tunnel: w165 -> [w182 w235]
                      tunnel: [w180 w235] -> w164
                      frame Default {
                        n91 = Increment(x=w198) -> (x+1=w199:i32)
                        n92 = Index Array(array=w197, index (col)=w198) -> (element=w196:string[])  [unwired: 1 in]
                        n93 = Index Array(array=w197, index (col)=w199) -> (element=w195:string[])  [unwired: 1 in]
                        n94 = Fract/Exp String To Number(string=w196) -> (number=w193:dbl[])  [unwired: 3 in, 1 out]
                        n95 = Fract/Exp String To Number(string=w195) -> (number=w194:dbl[])  [unwired: 3 in, 1 out]
                        n96 = case shown="False" "Switch off Tubing Correction?" {
                          tunnel: w194 -> [w220 _]
                          tunnel: w193 -> [w219 _]
                          tunnel: w192 -> [w218 _]
                          tunnel: w190 -> [w217 w234]
                          tunnel: [w216 w234] -> w183
                          tunnel: w188 -> [w215 w232]
                          tunnel: [w214 w232] -> w187
                          tunnel: w186 -> [w212 w233]
                          tunnel: [w213 w230] -> w181
                          frame False {
                            n97 = in-place {
                              in-place-border: w220 -> [w229]
                              in-place-border: w219 -> [w228]
                              in-place-border: w218 -> [w227]
                              in-place-border: w217 -> [w226]
                              in-place-border: [w225] -> w216
                              in-place-border: [w222] -> w213
                              in-place-border: w212 -> [w221]
                              n98 = in-place-array #1(w215, w212) -> (w224:T4)
                              n99 = call "EnFlo_TubingCorrection_Sub.vi"("Index"=w221, "Analysis Info cluster In"=w224, "Time Trace In"=w226, "Phase"=w229, "Gain"=w228, "Freq Hz"=w227) -> ("Time Trace out"=w225:T8, "Analysis Info cluster Out"=w223:T4)  [unwired: 2 in]
                              n100 = Unbundle By Name(w223) -> ("Device"=w222:string)
                              n101 = in-place-array #1(w223) -> (w214:T4[])  [unwired: 1 out]
                            }
                          }
                          frame True {
                            n102 = Index Array(array=w232, index=w233) -> (element=w231:T4)
                            n103 = Unbundle By Name(w231) -> ("Device"=w230:string)
                          }
                        }
                        n104 = case shown="Default" w181 {
                          tunnel: w185 -> [w201 w207]
                          tunnel: [w201 w206] -> w184
                          tunnel: w183 -> [_ w205]
                          tunnel: w182 -> [w200 w202]
                          tunnel: [w200 w203] -> w180
                          frame "7HP.vi" {
                          }
                          frame Default {
                            n105 = Unbundle By Name(w205) -> ("Eng Values"=w204:dbl[])
                            n106 = case shown="0" w202 {
                              tunnel: w207 -> [_ w211]
                              tunnel: [w208 w210] -> w206
                              tunnel: w204 -> [w208 w209]
                              frame 0 {
                              }
                              frame Default {
                                n107 = Add(x=w209, y=w211) -> (x+y=w210:dbl[])
                              }
                            }
                            n108 = Increment(x=w202) -> (x+1=w203:i32)
                          }
                        }
                      }
                      frame -1 {
                      }
                    }
                  }
                  n109 = Decrement(x="Reference Instrument") -> (x-1=w154:i32)
                  n110 = Divide(x=w151, y=w150) -> (x/y=w149:dbl[])
                }
                frame #2 {
                  w246 = 0.01 ("Timescale integral Estimate")
                  n111 = local read "Subtract Mode"() -> (w248:T2)
                  n112 = Index Array(array=w253, index=w240) -> (element=w247:T8)
                  n113 = Index Array(array=w250, index=w240) -> (element=w244:T4)
                  n114 = Bundle By Name(cluster=w244, "Timescale integral Estimate"=w246) -> (w245:T4)
                  n115 = case shown="\"Subtract Ref Channel\"" w248 {
                    tunnel: w252 -> [w255 w282 w351]
                    tunnel: w253 -> [w254 w274 w346]
                    tunnel: [w254 w273 w345] -> w243
                    tunnel: [w257 w281 w350] -> w241
                    tunnel: [w256 w280 w349] -> w242
                    tunnel: w251 -> [w258 w279 w348]
                    tunnel: w247 -> [_ w278 _]
                    tunnel: w245 -> [_ w277 w343]
                    tunnel: w250 -> [_ w276 w342]
                    tunnel: w246 -> [_ w275 w347]
                    tunnel: w249 -> [_ _ w344]
                    tunnel: w240 -> [_ w272 _]
                    tunnel: w240 -> [_ w271 _]
                    frame "Leave Data Alone" {
                      n116 = for {
                        tunnel: w254 -> [w269]
                        tunnel: w255 -> [w262] mode=indexing
                        tunnel: w258 -> [w263]
                        tunnel: [w260] -> w257 mode=indexing
                        tunnel: [w259] -> w256 mode=indexing
                        i -> [w261]
                        n117 = Index Array(array=w269, index=w262) -> (element=w270:T8)
                        n118 = Index Array(array=w263, index=w262) -> (element=w264:string)
                        n119 = Unbundle By Name(w270) -> ("Eng Values"=w268:dbl[])
                        n120 = call-poly <vilib>:"Mean.vi"("X"=w268) -> ("mean"=w259:dbl)  [unwired: 1 out]
                        n121 = Number To Decimal String(number=w261) -> (decimal integer string=w265:string)  [unwired: 1 in]
                        n122 = Number To Fractional String(number=w259, precision (6)=i16 3) -> (F-format string=w266:string)  [unwired: 2 in]
                        n123 = Build Array(w265, w264, w266) -> (w260:string[])
                      }
                    }
                    frame "Subtract Ref Channel" {
                      n124 = for {
                        tunnel: w282 -> [w286] mode=indexing
                        tunnel: [w287] -> w280 mode=indexing
                        tunnel: [w298] -> w281 mode=indexing
                        tunnel: w279 -> [w295]
                        tunnel: w278 -> [w293]
                        tunnel: w277 -> [w292]
                        tunnel: w276 -> [w291]
                        tunnel: w275 -> [w290]
                        shift-right: [w288] -> w273
                        shift-left: w274 -> [w289]
                        tunnel: w272 -> [w285]
                        tunnel: w271 -> [w283]
                        i -> [w297]
                        n125 = Equal?(x=w285, y=w286) -> (x = y?=w284:bool)
                        n126 = case shown="False" w284 {
                          tunnel: w293 -> [w309 _]
                          tunnel: w292 -> [w308 _]
                          tunnel: w291 -> [w307 _]
                          tunnel: w290 -> [w306 _]
                          tunnel: w289 -> [w305 w341]
                          tunnel: [w304 w341] -> w288
                          tunnel: [w303 0.0 ("mean")] -> w287
                          tunnel: w286 -> [w302 _]
                          tunnel: w283 -> [w301 _]
                          frame False {
                            n127 = in-place {
                              in-place-border: w309 -> [w313]
                              in-place-border: w308 -> [w321]
                              in-place-border: w302 -> [w318]
                              in-place-border: w307 -> [w327]
                              in-place-border: w306 -> [w326]
                              in-place-border: [w322] -> w303
                              in-place-border: w301 -> [w319]
                              n128 = in-place-array #2(w305, w302) -> (w312:T8)
                              n129 = Index Array(array=w327, index=w318) -> (element=w325:T4)
                              n130 = Bundle By Name(cluster=w325, "Timescale integral Estimate"=w326) -> (w320:T4)
                              n131 = call "Get Coincident Pairs.vi"("interp. method"=enum16{"nearest", "linear"}."linear", "Index2"=w318, "Index1"=w319, "Cluster 2"=w320, "Cluster 1"=w321) -> ("Pairs"=w316:cluster{"Cluster":T9, "Cluster":T9, dbl}, "Need to Update"=w317:bool)  [unwired: 5 in]
                              n132 = Unbundle By Name(w313) -> ("Eng Values"=w314:dbl[])
                              n133 = case shown="True" w317 {
                                tunnel: w316 -> [_ w336]
                                tunnel: w312 -> [w328 w331]
                                tunnel: [w329 w333] -> w315
                                tunnel: w314 -> [w329 w335]
                                tunnel: [w328 w332] -> w311
                                frame False {
                                }
                                frame True {
                                n134 = Unbundle(w336) -> ("Cluster"=w334:T9, "Cluster"=w330:T9)  [unwired: 1 out]
                                n135 = call "Index Coincident Pairs.vi"("Interpolation method"=w330, "Time Cluster 1"=w331) -> ("Time Cluster 1 Out"=w332:T8)  [unwired: 1 in]
                                n136 = call "Select indexed values.vi"("Cluster"=w334, "Values"=w335) -> ("Values Out"=w333:dbl[])  [unwired: 1 in]
                                }
                              }
                              n137 = in-place {
                                in-place-border: w315 -> [w339]
                                in-place-border: [w337] -> w323
                                n138 = in-place-cluster #3(w311) -> ("Eng Values"=w338:dbl[])
                                n139 = Subtract(x=w338, y=w339) -> (x-y=w337:dbl[])
                                n140 = in-place-cluster #3("Eng Values"=w337) -> (w324:T8)
                              }
                              n141 = call-poly <vilib>:"Mean.vi"("X"=w323) -> ("mean"=w322:dbl)  [unwired: 1 out]
                              n142 = in-place-array #2(w324) -> (w304:T8[])  [unwired: 1 out]
                            }
                          }
                          frame True {
                          }
                        }
                        n143 = Index Array(array=w295, index=w286) -> (element=w294:string)
                        n144 = Number To Decimal String(number=w297) -> (decimal integer string=w296:string)  [unwired: 1 in]
                        n145 = Number To Fractional String(number=w287, precision (6)=i16 3) -> (F-format string=w299:string)  [unwired: 2 in]
                        n146 = Build Array(w296, w294, w299) -> (w298:string[])
                      }
                    }
                    frame "Subtract Instantaneous Average of All Chs" {
                      n147 = for {
                        tunnel: w351 -> [w352] mode=indexing
                        tunnel: [w356] -> w349 mode=indexing
                        tunnel: [w364] -> w350 mode=indexing
                        tunnel: w348 -> [w361]
                        tunnel: w347 -> [w359]
                        shift-right: [w357] -> w345
                        shift-left: w346 -> [w358]
                        tunnel: w344 -> [w355]
                        tunnel: w343 -> [w354]
                        tunnel: w342 -> [w353]
                        i -> [w363]
                        n148 = in-place {
                          in-place-border: w352 -> [_]
                          in-place-border: w359 -> [_]
                          in-place-border: [w373] -> w356
                          in-place-border: w355 -> [w375]
                          in-place-border: w354 -> [w372]
                          in-place-border: w353 -> [w370]
                          in-place-border: w352 -> [w369]
                          n149 = in-place-array #4(w358, w352) -> (w376:T8)
                          n150 = Index Array(array=w370, index=w369) -> (element=w368:T4)
                          n151 = Unbundle By Name(w368) -> ("Device"=w367:string, "Inst type"=w371:T5)
                          n152 = case shown="\"Pitot-static tube\"" w371 {
                            tunnel: w376 -> [w381 w405]
                            tunnel: w375 -> [w380 w394]
                            tunnel: [w379 w404] -> w374
                            tunnel: [w378 w403] -> w373
                            tunnel: w372 -> [_ _]
                            tunnel: w368 -> [_ w393]
                            tunnel: w367 -> [w377 _]
                            frame Default {
                              n153 = case shown="Default" w377 {
                                tunnel: w381 -> [w384 w388]
                                tunnel: w380 -> [_ w387]
                                tunnel: [w384 w386] -> w379
                                tunnel: [w382 w385] -> w378
                                frame "7HP.vi" {
                                n154 = Unbundle By Name(w384) -> ("Eng Values"=w383:dbl[])
                                n155 = call-poly <vilib>:"Mean.vi"("X"=w383) -> ("mean"=w382:dbl)  [unwired: 1 out]
                                }
                                frame Default {
                                n156 = in-place {
                                in-place-border: w387 -> [w392]
                                in-place-border: [w389] -> w385
                                n157 = in-place-cluster #5(w388) -> ("Eng Values"=w391:dbl[])
                                n158 = Subtract(x=w391, y=w392) -> (x-y=w390:dbl[])
                                n159 = call-poly <vilib>:"Mean.vi"("X"=w390) -> ("mean"=w389:dbl)  [unwired: 1 out]
                                n160 = in-place-cluster #5("Eng Values"=w390) -> (w386:T8)
                                }
                                }
                              }
                            }
                            frame "Pitot-static tube" {
                              n161 = Unbundle By Name(w405) -> ("Voltage"=w396:dbl[])
                              n162 = Unbundle By Name(w393) -> ("Calib Constants"=w400:dbl[])
                              n163 = call "Offset Channel Index.vi"() -> ("index"=w399:i32)
                              n164 = Subtract(x=w396, y=w394) -> (x-y=w395:dbl[])
                              n165 = global read "Meas_global.vi" "Abs Press (mbar)"() -> (w402:dbl)
                              n166 = Index Array(array=w400, index=w399) -> (element=w398:dbl)
                              n167 = call-poly <vilib>:"Mean.vi"("X"=w395) -> ("mean"=w403:dbl)  [unwired: 1 out]
                              n168 = global read "Meas_global.vi" "Temp"() -> (w401:dbl)
                              n169 = call "Pitot-static_to_Velocity.vi"("Pressure Trans voltage"=w395, "Atmos Press mbar  (1000)"=w402, "Temp  C  (20)"=w401, "Pressure Trans Calib const"=w400, "Mano Zero"=w398) -> ("Velocity (m/s)"=w397:dbl[])  [unwired: 1 in, 2 out]
                              n170 = Bundle By Name(cluster=w405, "Voltage"=w395, "Eng Values"=w397) -> (w404:T8)
                            }
                          }
                          n171 = in-place-array #4(w374) -> (w357:T8[])  [unwired: 1 out]
                        }
                        n172 = Index Array(array=w361, index=w352) -> (element=w360:string)
                        n173 = Number To Decimal String(number=w363) -> (decimal integer string=w362:string)  [unwired: 1 in]
                        n174 = Number To Fractional String(number=w356, precision (6)=i16 3) -> (F-format string=w365:string)  [unwired: 2 in]
                        n175 = Build Array(w362, w360, w365) -> (w364:string[])
                      }
                    }
                  }
                }
                frame #3 {
                  n176 = case shown="\"Correlate with Ref Channel\"" "Correlation Mode" {
                    tunnel: w421 -> [_ w441]
                    tunnel: w420 -> [_ w440]
                    tunnel: w419 -> [_ w427]
                    tunnel: w418 -> [_ w435]
                    tunnel: w417 -> [w425 w434]
                    tunnel: [w425 w433] -> w416
                    tunnel: [w424 w432] -> w414
                    tunnel: w413 -> [w424 _]
                    tunnel: [w423 "Correlation Coeff"] -> w412
                    tunnel: [w423 "Corr Coeff"] -> w408
                    tunnel: [w422 w428] -> w407
                    tunnel: w406 -> [w422 w429]
                    frame "Leave Data Alone" {
                      w423 = "Pressures"
                    }
                    frame "Correlate with Ref Channel" {
                      w438 = 0.01 ("Timescale integral Estimate")
                      n177 = Index Array(array=w435, index=w427) -> (element=w439:T8)
                      n178 = Index Array(array=w440, index=w427) -> (element=w436:T4)
                      n179 = Bundle By Name(cluster=w436, "Timescale integral Estimate"=w438) -> (w437:T4)
                      n180 = for {
                        tunnel: w441 -> [w451] mode=indexing
                        tunnel: w435 -> [w467]
                        tunnel: w439 -> [w450]
                        tunnel: w437 -> [w454]
                        tunnel: w440 -> [w465]
                        tunnel: w438 -> [w464]
                        shift-right: [w461] -> w433
                        shift-left: w434 -> [w462]
                        tunnel: [w460] -> w432 mode=indexing
                        tunnel: w429 -> [w459] mode=indexing
                        tunnel: [w455] -> w428 mode=indexing
                        tunnel: w427 -> [w452]
                        tunnel: enum16{"nearest", "linear"}."linear" ("interp. method") -> [w442]
                        n181 = Index Array(array=w465, index=w451) -> (element=w463:T4)
                        n182 = Index Array(array=w467, index=w451) -> (element=w449:T8)
                        n183 = Unbundle By Name(w450) -> ("Eng Values"=w447:dbl[])
                        n184 = Unbundle By Name(w449) -> ("Eng Values"=w445:dbl[])
                        n185 = Bundle By Name(cluster=w463, "Timescale integral Estimate"=w464) -> (w453:T4)
                        n186 = call "Get Coincident Pairs.vi"("interp. method"=w442, "Index2"=w451, "Index1"=w452, "Cluster 2"=w453, "Cluster 1"=w454) -> ("Pairs"=w443:cluster{"Cluster":T9, "Cluster":T9, dbl}, "Need to Update"=w448:bool)  [unwired: 5 in]
                        n187 = case shown="True" w448 {
                          tunnel: w447 -> [w469 w473]
                          tunnel: [w469 w470] -> w446
                          tunnel: w445 -> [w468 w472]
                          tunnel: [w468 w471] -> w444
                          tunnel: w443 -> [_ w476]
                          frame False {
                          }
                          frame True {
                            n188 = Unbundle(w476) -> ("Cluster"=w474:T9, "Cluster"=w475:T9)  [unwired: 1 out]
                            n189 = call "Select indexed values.vi"("Cluster"=w474, "Values"=w473) -> ("Values Out"=w470:dbl[])  [unwired: 1 in]
                            n190 = call "Select indexed values.vi"("Cluster"=w475, "Values"=w472) -> ("Values Out"=w471:dbl[])  [unwired: 1 in]
                          }
                        }
                        n191 = call <vilib>:"Correlation Coefficient.vi"("Y"=w444, "X"=w446) -> ("correlation coefficient r"=w460:dbl)  [unwired: 8 in, 1 out]
                        n192 = Number To Fractional String(number=w460, precision (6)=i16 3) -> (F-format string=w456:string)  [unwired: 2 in]
                        n193 = in-place {
                          in-place-border: w456 -> [w477]
                          n194 = in-place-array #6(w462, w451) -> (w483:T4)
                          n195 = Unbundle By Name(w483) -> ("Inst name"=w482:string)
                          n196 = Format Into String(format string="%s:Correlation Coeff:With Ref", w482) -> (resulting string=w480:string)  [unwired: 2 in, 1 out]
                          n197 = Build Array(w480) -> (w479:string[])
                          n198 = Build Array(w477) -> (w478:string[])
                          n199 = call "Update Metadata channels.vi"("Metadata Values"=w478, "Metadata Names"=w479, "Analysis info Cluster in"=w483) -> ("Analysis info Cluster out"=w484:T4)
                          n200 = in-place-array #6(w484) -> (w461:T4[])  [unwired: 1 out]
                        }
                        n201 = Array Subset(array=w459, length=2) -> (w457:string[])  [unwired: 1 in]
                        n202 = Build Array (concatenate)(w457, w456) -> (w455:string[])
                      }
                    }
                  }
                  "?" <- w414
                  "Correlation Coefficients" <- w407
                  n203 = property class="WFGraph (strict)"("YScale.NameLbl.Text"=w412) -> ()  [unwired: 2 in, 2 out]
                  n204 = global write "Meas_global.vi" "Analysis Info cluster"(w416) -> ()
                  n205 = Build Array("Ch No", "Channel Name", w408) -> (w411:string[])
                  n206 = property on="Correlation Coefficients" class="Tbl (strict)"("Column Headers[]"=w411) -> ()  [unwired: 2 in, 2 out]
                }
                frame #4 {
                  n207 = Index Array(array=w501) -> (element=w488:i32)  [unwired: 1 in]
                  n208 = call "Get Time Trace.vi"("Channel Index"=w488) -> ("Time (s)"=w487:dbl[])  [unwired: 1 out]
                  n209 = global read "Meas_global.vi" "Time Array Index"() -> (w489:i32[])
                  n210 = Index Array(array=w487, index #1=1 ("index"), index #2=0 ("index")) -> (element #1=w494:dbl, element #2=w495:dbl)
                  n211 = Subtract(x=w494, y=w495) -> (x-y=w493:dbl)
                  n212 = global read "Meas_global.vi" "Unique Times"() -> (w485:cluster{"Time (s)":dbl[]}[])
                  n213 = Reciprocal(x=w493) -> (1/x=w492:dbl)
                  n214 = Divide(x=w492, y="Desired Freq Hz") -> (x/y=w499:dbl)
                  n215 = Round To Nearest(number=w499) -> (nearest integer value=w498:dbl)
                  n216 = To Long Integer(number=w498) -> (32bit integer=w490:i32)
                  "Averaging samples" <- w490
                  n217 = for {
                    tunnel: w501 -> [w509] mode=indexing
                    tunnel: w490 -> [w511]
                    shift-right: [w513] -> w502
                    shift-left: w500 -> [w512]
                    tunnel: w489 -> [w510]
                    shift-right: [w505] -> _
                    shift-left: _ -> [w506]
                    shift-right: [w503] -> _
                    shift-left: -1 ("Numeric") -> [w508]
                    tunnel: w485 -> [w504]
                    n218 = in-place {
                      in-place-border: w511 -> [w523]
                      n219 = in-place-array #7(w512, w509) -> (w521:T8)
                      n220 = in-place {
                        in-place-border: w523 -> [w524]
                        n221 = in-place-cluster #8(w521) -> ("Weighting"=w530:dbl[], "Voltage"=w529:dbl[], "Eng Values"=w528:dbl[])
                        n222 = call "Downsampler.vi"("Input Array"=w530, "Averaging samples"=w524) -> ("Downsampled Array"=w525:dbl[])  [unwired: 1 out]
                        n223 = call "Downsampler.vi"("Input Array"=w529, "Averaging samples"=w524) -> ("Downsampled Array"=w526:dbl[])  [unwired: 1 out]
                        n224 = call "Downsampler.vi"("Input Array"=w528, "Averaging samples"=w524) -> ("Downsampled Array"=w527:dbl[])  [unwired: 1 out]
                        n225 = in-place-cluster #8("Weighting"=w525, "Voltage"=w526, "Eng Values"=w527) -> (w522:T8)
                      }
                      n226 = in-place-array #7(w522) -> (w513:T8[])  [unwired: 1 out]
                    }
                    n227 = Index Array(array=w510, index=w509) -> (element=w503:i32)
                    n228 = Equal?(x=w503, y=w508) -> (x = y?=w507:bool)
                    n229 = case shown="False" w507 {
                      tunnel: w511 -> [w519 _]
                      tunnel: [w518 w520] -> w505
                      tunnel: w506 -> [_ w520]
                      tunnel: w504 -> [w517 _]
                      tunnel: w503 -> [w514 _]
                      frame False {
                        n230 = Index Array(array=w517, index=w514) -> (element=w516:cluster{"Time (s)":dbl[]})
                        n231 = Unbundle(w516) -> ("Time (s)"=w515:dbl[])
                        n232 = call "Downsampler.vi"("Input Array"=w515, "Averaging samples"=w519) -> ("Downsampled Array"=w518:dbl[])  [unwired: 1 out]
                      }
                      frame True {
                      }
                    }
                    n233 = call "Update Time Trace.vi"("Channel Index"=w509, "Time (s)"=w505) -> ()  [unwired: 1 in]
                  }
                  n234 = global write "Meas_global.vi" "Time Trace"(w502) -> ()
                }
                frame #5 {
                  n235 = global read "Meas_global.vi" "Post Process"() -> (w531:T10)
                  n236 = case shown="\"Take New Data\"" w531 {
                    frame "Take New Data" {
                      n237 = global read "Meas_global.vi" "Raw data file"() -> (w538:path)
                      n238 = call "Get Raw Data Folder.vi"("Raw data file"=w538) -> ("Main Raw Data Folder"=w537:path)
                      n239 = Build Path(base path=w537, name or relative path="Extra Info") -> (appended path=w539:path)
                      n240 = Strip Path(path="Select Freq Calib file") -> (name=w536:string)  [unwired: 1 out]
                      n241 = Build Path(base path=w539, name or relative path=w536) -> (appended path=w533:path)
                      n242 = call "Create_directory_path.vi"("Path name"=w533) -> ("Path name Out"=w532:path)  [unwired: 2 in, 1 out]
                      n243 = call "Does_file_exist_(simple).vi"("Pathname"=w532) -> ("exists?"=w535:bool)
                      n244 = case shown="False" w535 {
                        tunnel: "Select Freq Calib file" -> [w542 _]
                        tunnel: w532 -> [w541 _]
                        frame False {
                          n245 = Copy(10:w541, 11:w542) -> ()  [unwired: 3 in, 3 out]
                        }
                        frame True {
                        }
                      }
                    }
                    frame "Post Process Raw Data File" {
                    }
                  }
                }
                frame #6 {
                  n246 = case shown="True" w543 {
                    tunnel: w545 -> [_ w549]
                    tunnel: w544 -> [_ w546]
                    frame False {
                    }
                    frame True {
                      n247 = global read "Meas_global.vi" "New Setup String"() -> (w547:string)
                      n248 = call "Replace_data_in_Label_str.vi"("New data string"=w546, "Input string"=w547, "Variable name"=w549) -> ("Appended string"=w548:string)
                      n249 = global write "Meas_global.vi" "New Setup String"(w548) -> ()
                    }
                  }
                }
              }
            }
          }
        }
        frame #4 {
          n250 = case shown="True" w554 {
            tunnel: w553 -> [_ w562]
            tunnel: w552 -> [_ w561]
            tunnel: w551 -> [_ w560]
            tunnel: w550 -> [_ _]
            frame False {
              # "All"
              # "Hz"
            }
            frame True {
              n251 = local read "Select Freq Calib file"() -> (w556:path)
              n252 = call "Save Plugin Setup String.vi"("Plug In Pathname"=w561, "Setup String to Save"=w560, "PlugIn Label"=w562) -> ("Meas Setup File"=w555:bool, "Raw Data File Written to"=w559:path[])
              n253 = Strip Path(path=w556) -> (name=w558:string)  [unwired: 1 out]
              n254 = for {
                tunnel: w559 -> [w570] mode=indexing
                tunnel: w558 -> [w569]
                shift-right: [w565] -> _
                shift-left: path[] [] -> [w567]
                tunnel: w556 -> [w563]
                tunnel: w555 -> [w564]
                n255 = case shown="True" w564 {
                  tunnel: w570 -> [w573 _]
                  tunnel: w569 -> [w572 _]
                  tunnel: [w571 w578] -> w566
                  tunnel: w563 -> [_ w579]
                  frame False {
                    n256 = call "Get Raw Data Folder.vi"("Raw data file"=w573) -> ("Main Raw Data Folder"=w575:path)
                    n257 = Build Path(base path=w575, name or relative path="Extra Info") -> (appended path=w576:path)
                    n258 = Build Path(base path=w576, name or relative path=w572) -> (appended path=w574:path)
                    n259 = call "Create_directory_path.vi"("Path name"=w574) -> ("Path name Out"=w571:path)  [unwired: 2 in, 1 out]
                  }
                  frame True {
                    n260 = call "Current_Filepath.vi"("Short_Name"="Cal" ("Data Type"), "Filename in"=w579, "Data Type"="Calibrations") -> ("Filename Out"=w578:path)  [unwired: 1 in, 1 out]
                  }
                }
                n261 = Search 1D Array(1D array=w567, element=w566) -> (index of element=w568:i32)  [unwired: 1 in]
                n262 = case shown="-1" w568 {
                  tunnel: w567 -> [w582 w587]
                  tunnel: w566 -> [_ w584]
                  tunnel: [w582 w586] -> w565
                  tunnel: w563 -> [_ w583]
                  frame 0, Default {
                  }
                  frame -1 {
                    n263 = Build Array (concatenate)(w587, w584) -> (w586:path[])
                    n264 = call "Does_file_exist_(simple).vi"("Pathname"=w584) -> ("exists?"=w585:bool)
                    n265 = case shown="False" w585 {
                      tunnel: w584 -> [w589 _]
                      tunnel: w583 -> [w588 _]
                      frame False {
                        n266 = Copy(10:w589, 11:w588) -> ()  [unwired: 3 in, 3 out]
                      }
                      frame True {
                      }
                    }
                  }
                }
              }
            }
          }
        }
      }
    }
    frame True {
    }
  }
